vi "Stop Core.vi"(10 "final error code":i32, 11 "Actor_Controller_Template in":refnum<class "Actor_Controller_Template.lvclass">) -> (3 "Actor_Controller_Template out":refnum<class "Actor_Controller_Template.lvclass">)   [LabVIEW 2020, in "Actor_Controller_Template.lvlib" / "Actor_Controller_Template.lvclass"]
doc: "(<B>Filename</B>: Actor Framework.lvlib:Actor.lvclass:Stop Core.vi)\n\nDefines what the actor does before it stops. Use the <B>final error code</B> input to determine whether the actor shut down in response to an error.\n\nBy default, this method passes the Stop message along to all auto-stop nested actors. A descendant class may override this method to define additional behavior, such as shutting down any processes the actor initiated in its override of the Actor Core method."
uses:
  Actor_Controller_Template.lvclass
  Actor_Controller_Template.lvclass/Actor_Controller_Template.ctl
  <vilib>/ActorFramework/Stop Msg/Stop Msg.lvclass/Stop Msg.ctl
  <vilib>/ActorFramework/Message Enqueuer/Message Enqueuer.lvclass/Message Enqueuer.ctl
  <vilib>/ActorFramework/Stop Msg/Send Emergency Stop.vi
  <vilib>/ActorFramework/Stop Msg/Send Normal Stop.vi
  <vilib>/ActorFramework/Message Enqueuer/Enqueue Critical.vi
  <vilib>/ActorFramework/Message Enqueuer/Enqueue.vi
  <vilib>/ActorFramework/Stop Msg/Stop Msg.lvclass
  C:/Program Files/National Instruments/LabVIEW 2020/vi.lib/ActorFramework/Message/Message.lvclass
  <vilib>/ActorFramework/Message Priority Queue/Priority Enqueue.vi
  <vilib>/ActorFramework/Actor/Actor.lvclass
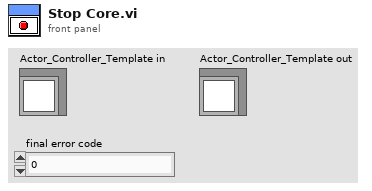
[diagram p1: front panel]
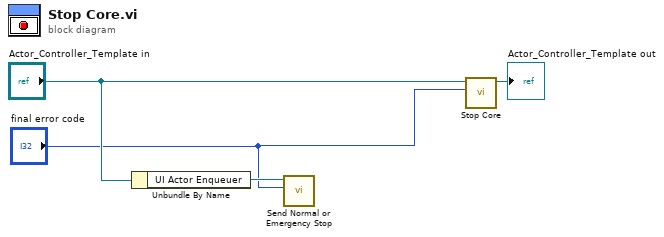
[diagram p0: block diagram]
diagram:
  n1 = Unbundle By Name("Actor_Controller_Template in") -> ("UI Actor Enqueuer"=w2:refnum<class "Message Enqueuer.lvclass">)
  n2 = call <vilib>:"Send Normal or Emergency Stop.vi"("final error code"="final error code", "Message Enqueuer"=w2) -> ()  [unwired: 9 in, 1 out]
  n3 = call-parent "Stop Core.vi"("final error code"="final error code", "Actor in"="Actor_Controller_Template in") -> ("Actor out"=→"Actor_Controller_Template out":refnum<class "Actor_Controller_Template.lvclass">)  [unwired: 9 in]
